vi "SACB - 2.vi"(6 "RH?":bool, 7 "Command":enum16{"Create", "Read", "Close"}(ring), 8 "Error In":errorcluster) -> (0 "Error Out":errorcluster, 3 "Digital Inputs":T1)   [LabVIEW 2017]
uses:
  <vilib>/Modbus/master/Modbus Master.lvclass
  <vilib>/Modbus/master/Create Master Instance (TCP).vi
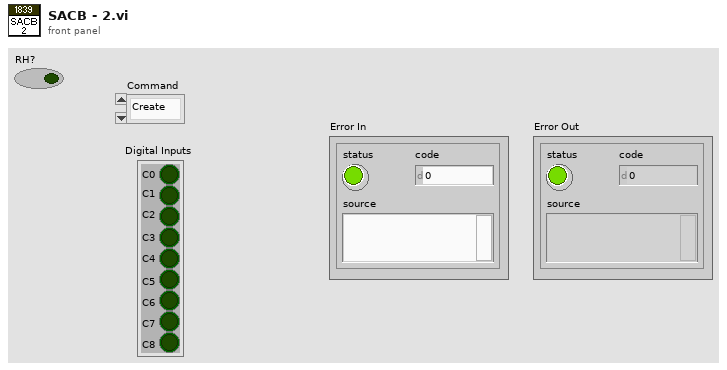
[diagram p1: front panel]
types:
  T1 = cluster{"C0":bool, "C1":bool, "C2":bool, "C3":bool, "C4":bool, "C5":bool, "C6":bool, "C7":bool, "C8":bool}
  T2 = cluster{"Boolean array[0]":bool, "Boolean array[1]":bool, "Boolean array[2]":bool, "Boolean array[3]":bool, "Boolean array[4]":bool, "Boolean array[5]":bool, "Boolean array[6]":bool, "Boolean array[7]":bool, "Boolean array[8]":bool}
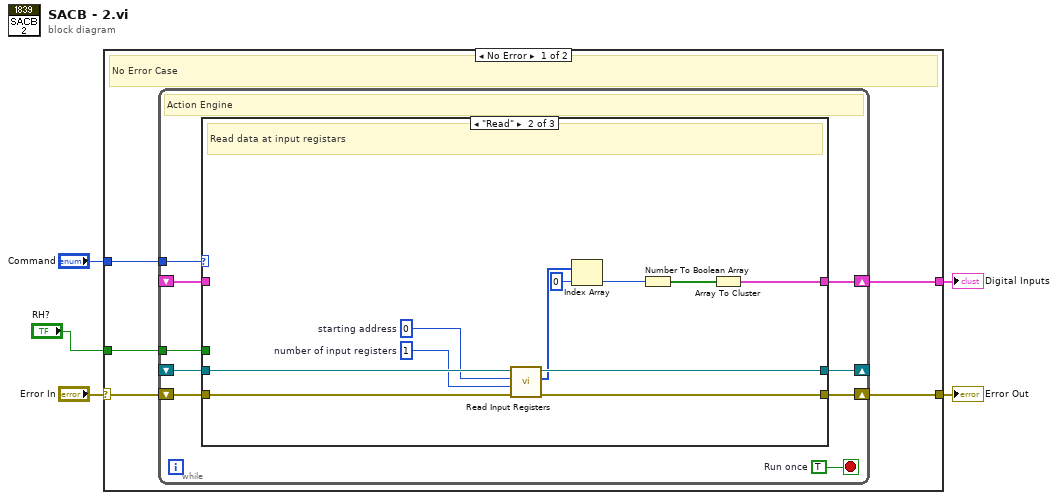
[diagram p0: block diagram]
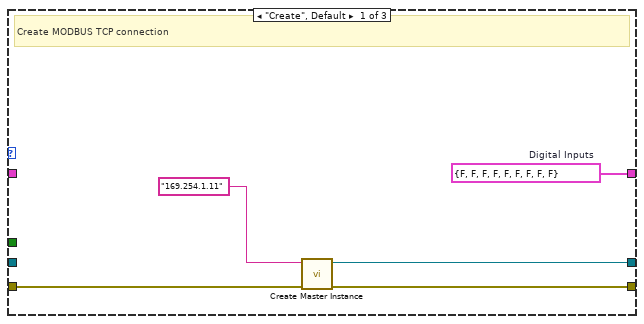
[diagram p2: hidden frame]
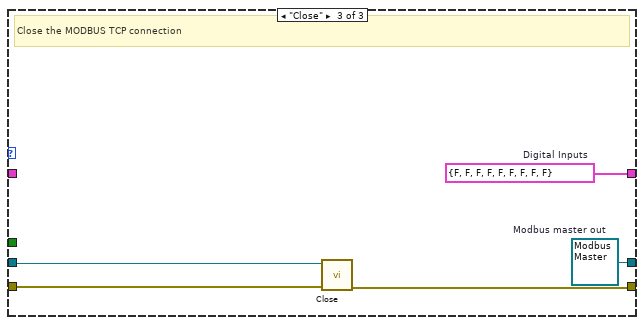
[diagram p3: hidden frame]
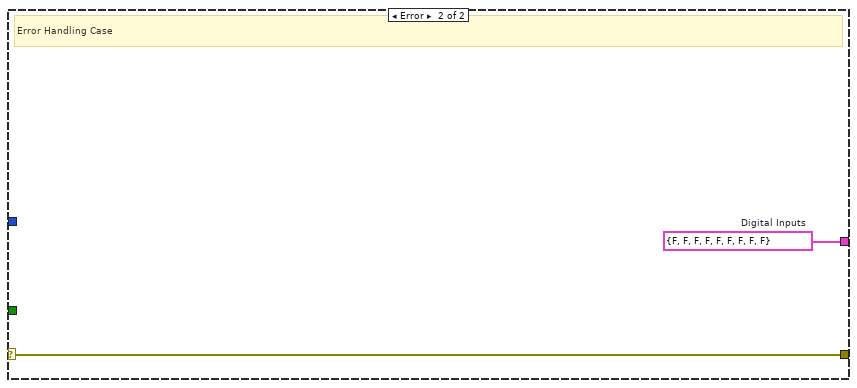
[diagram p4: hidden frame]
diagram:
  n1 = case shown="No Error" "Error In" {
    selector: "Error In" -> [w9 w42]
    tunnel: [w10 w42] -> w4
    tunnel: "Command" -> [w8 _]
    tunnel: [w7 w41] -> w2
    tunnel: "RH?" -> [w6 _]
    frame No Error {
      # "No Error Case"
      n2 = while {
        tunnel: w8 -> [w17]
        shift-right: [w19] -> w10
        shift-left: w9 -> [w18]
        shift-right: [w15] -> _
        shift-left: _ -> [w14]
        shift-right: [w13] -> w7
        shift-left: _ -> [w12]
        tunnel: w6 -> [w11]
        stop <- w16 stop-if-true
        w16 = TRUE  # Run once
        # "Action Engine"
        n3 = case shown="\"Read\"" w17 {
          tunnel: [w24 w34 w39] -> w19
          tunnel: w18 -> [w23 w35 w40]
          tunnel: [w22 w33 w37] -> w15
          tunnel: w14 -> [_ w32 w38]
          tunnel: [w21 w25 w36] -> w13
          tunnel: w12 -> [_ _ _]
          tunnel: w11 -> [_ _ _]
          frame "Create", Default {
            w21 = T1 {"C0"=FALSE, "C1"=FALSE, "C2"=FALSE, "C3"=FALSE, "C4"=FALSE, "C5"=FALSE, "C6"=FALSE, "C7"=FALSE, "C8"=FALSE}  # Digital Inputs
            # "Create MODBUS TCP connection"
            n4 = call-poly <vilib>:"Create Master Instance.vi"("error in (no error)"=w23, "address"="169.254.1.11") -> ("error out"=w24:errorcluster, "TCP master instance"=w22:refnum<class "Modbus Master.lvclass">)  [unwired: 8 in]
          }
          frame "Read" {
            w30 = u16 1  # number of input registers
            w31 = u16 0  # starting address
            # "Read data at input registars"
            n5 = call-dynamic "Read Input Registers.vi"("error in (no error)"=w35, "number of input registers"=w30, "starting address"=w31, "Modbus master in"=w32) -> ("error out"=w34:errorcluster, "register values"=w27:u16[], "Modbus master out"=w33:refnum<class "Modbus Master.lvclass">)  [unwired: 5 in]
            n6 = Index Array "Index Array"(array=w27, index=0) -> (element=w28:u16)
            n7 = Number To Boolean Array(number=w28) -> (Boolean array=w29:bool[])
            n8 = Array To Cluster(array=w29) -> (cluster=w25:T2)
          }
          frame "Close" {
            w36 = T1 {"C0"=FALSE, "C1"=FALSE, "C2"=FALSE, "C3"=FALSE, "C4"=FALSE, "C5"=FALSE, "C6"=FALSE, "C7"=FALSE, "C8"=FALSE}  # Digital Inputs
            w37 = refnum<class "Modbus Master.lvclass"> refnum  # Modbus master out
            # "Close the MODBUS TCP connection"
            n9 = call-dynamic "Close.vi"("error in (no error)"=w40, "Modbus master in"=w38) -> ("error out"=w39:errorcluster)  [unwired: 9 in]
          }
        }
      }
    }
    frame Error {
      w41 = T1 {"C0"=FALSE, "C1"=FALSE, "C2"=FALSE, "C3"=FALSE, "C4"=FALSE, "C5"=FALSE, "C6"=FALSE, "C7"=FALSE, "C8"=FALSE}  # Digital Inputs
      # "Error Handling Case"
    }
  }
  "Error Out" <- w4
  "Digital Inputs" <- w2
